vi "GetLeCroy_SaveToFile_25_AVG.vi"(1 "File Array":string[](array[string]), 2 "lines per plane":i32, 5 "Digitizer Settings":T1={"Digitizer delay (us) "=0.0, "rf points per line"=2048, "lines per plane"=128, "Samp Rate (Hz)"=100000000.0, "Additional dig delay (us)"=0.0, "Voltage Scale"=0.4, "Pre-Looks"=0, "Offset delay (us)"=0.0, "bits A/D"=8, "Avg Num"=1, "DigTimeOut"=5.0, "Rel Dig Delay"=0.0, "Dig Ch"=0, "LeCroyCluster"={"LeCroy Channels"=[TRUE, FALSE, FALSE, FALSE], "LC read pt offset"=0.0, "Sweep Avg"=FALSE}, "Main Digitizer"=enum."NI Digitizer", "Dig Config"=enum."Single channel", "Digitizer ID Cluster"={"Acqiris/Alazar/SP ID"=[], "NI Instr Handles"=[], "LeCroy VISA"="", "GaGe Handle"={"Handle"=0, "Sample size"=0, "Resolution"=0, "Offset"=0, "Channels"=0, "Boards"=0}, "ATS Ref"="ATS9350", "Acqiris Address"=["PCI::INSTR0"], "ADQRef"=refnum, "adq_cu_ptr"=refnum}, "Trigger Settings"={"Trig Source"=1, "Trig Coupling"=0, "Trig Slope"=0, "Level (mV)"=1500.0}, "Bulk Acq"=FALSE, "Bulk Start Indexes"=[], "Data Ref RF"=refnum, "NI ID/Channel"=[], "Total Dig CH"=1, "Xtra Ann Trig delay (us)"=10.0, "Fix Z Delay?"=FALSE, "One Way Transmission?"=FALSE, "Data Ref Log"=refnum} {"Trigger Settings"."Trig Slope" items=["Positive", "Negative"]; "Trigger Settings"."Level (mV)" format="%.2f"; "Trigger Settings"."Trig Coupling" items=["DC 1 MOhm", "AC 1 MOhm", "DC 50 Ohm", "AC 50 Ohm"]; "Trigger Settings"."Trig Source" items=["Chan 1", "External"]; "Rel Dig Delay" format="%.2f"; "DigTimeOut" format="%.2f"; "Avg Num" min=1; "Offset delay (us)" format="%.2f"; "Additional dig delay (us)" format="%.2f"; "Digitizer delay (us)" format="%.2f"}, 11 "errorin":errorcluster) -> (3 "Gain Array":T5(array[cluster]), 6 "VGain (dB)":dbl, 8 "data out":i16[][][](array[numeric]), 14 "Raw VGain (scale)":dbl, 15 "error out":errorcluster)   [LabVIEW 2022 SP3]
uses:
  -DigitizerRoutines/DigitizerSettings.ctl
  -DigitizerRoutines/Digitizer.ctl
  -DigitizerRoutines/DigConfig.ctl
  -DigitizerRoutines/DigitizerID.ctl
  C:/Windows/System32/ADQAPI_dotNet_helper.dll
panel:
  out "read time":u32
  out "save time":u32
  out "Numeric":i32
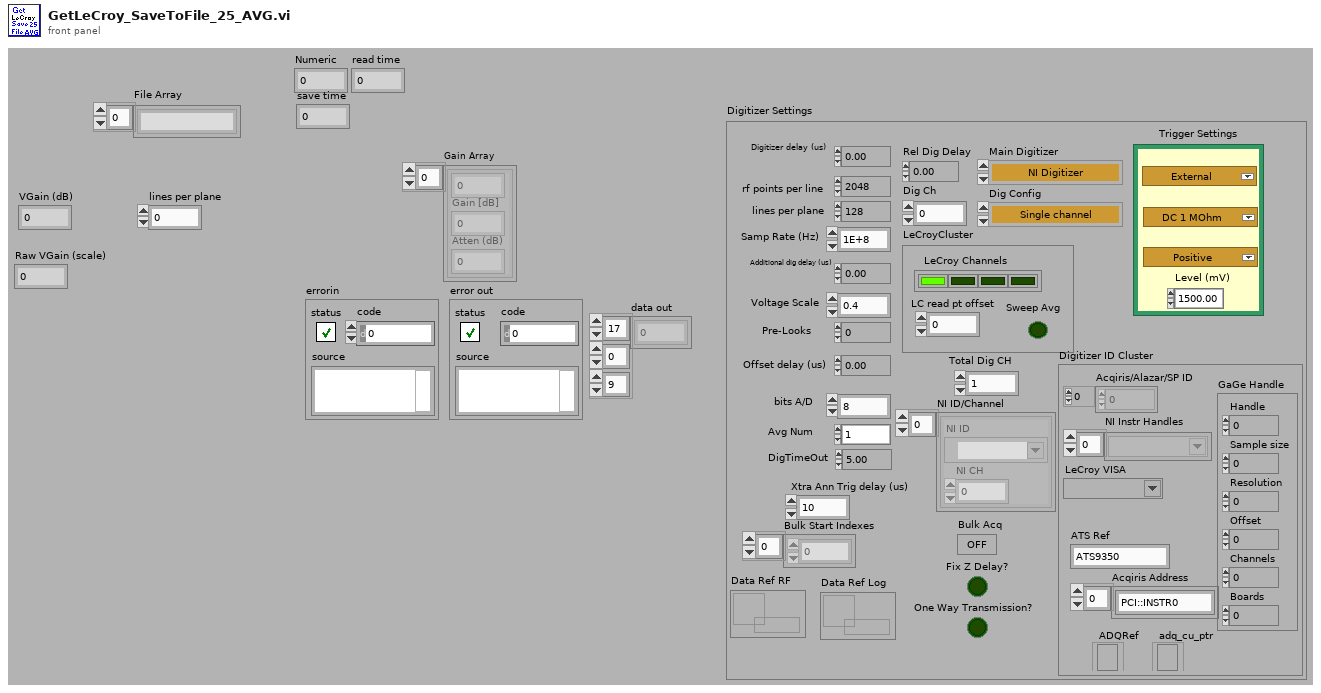
[diagram p1: front panel]
types:
  T1 = typedef "DigitizerSettings.ctl" = cluster{"Digitizer delay (us) ":dbl, "rf points per line":i32, "lines per plane":i32, "Samp Rate (Hz)":dbl, "Additional dig delay (us)":dbl, "Voltage Scale":dbl, "Pre-Looks":i32, "Offset delay (us)":dbl, "bits A/D":i8, "Avg Num":i32, "DigTimeOut":sgl, "Rel Dig Delay":sgl, "Dig Ch":i32, "LeCroyCluster":cluster{"LeCroy Channels":bool[], "LC read pt offset":dbl, "Sweep Avg":bool}, "Main Digitizer":T2, "Dig Config":T3, "Digitizer ID Cluster":T4, "Trigger Settings":cluster{"Trig Source":u16, "Trig Coupling":u16, "Trig Slope":u16, "Level (mV)":dbl}, "Bulk Acq":bool, "Bulk Start Indexes":i32[], "Data Ref RF":refnum<data-value>, "NI ID/Channel":cluster{"NI ID":refnum<k15>, "NI CH":i32}[], "Total Dig CH":i32, "Xtra Ann Trig delay (us)":dbl, "Fix Z Delay?":bool, "One Way Transmission?":bool, "Data Ref Log":refnum<data-value>}
  T2 = typedef "Digitizer.ctl" = enum16{"Acqiris Digitizer", "NI Digitizer", "LeCroy", "GaGe", "AlazarTech", "No Digitizer", "Teledyne"}
  T3 = typedef "DigConfig.ctl" = enum16{"Single channel", "2 Chans w/ 2 Acqiris", "2 Chans w/ 1 Acqiris", "5-CH Pulser New", "5-CH pulser w/ ann array", "5-pass style ann array", "Empty"}
  T4 = typedef "DigitizerID.ctl" = cluster{"Acqiris/Alazar/SP ID":u32[], "NI Instr Handles":refnum<k15>[], "LeCroy VISA":refnum<visa-resource-name>, "GaGe Handle":cluster{"Handle":u32, "Sample size":u32, "Resolution":i32, "Offset":i32, "Channels":u32, "Boards":u32}, "ATS Ref":string, "Acqiris Address":string[], "ADQRef":refnum<k24>, "adq_cu_ptr":refnum<k24>}
  T5 = cluster{sgl, "Gain [dB]  ":sgl, "Atten (dB)":sgl}[]
  T6 = cluster{"wfm":i16[][], "max queue size (-1, unlimited)":i32}
  T7 = cluster{sgl, "Gain [dB]  ":sgl, "Atten (dB)":sgl}
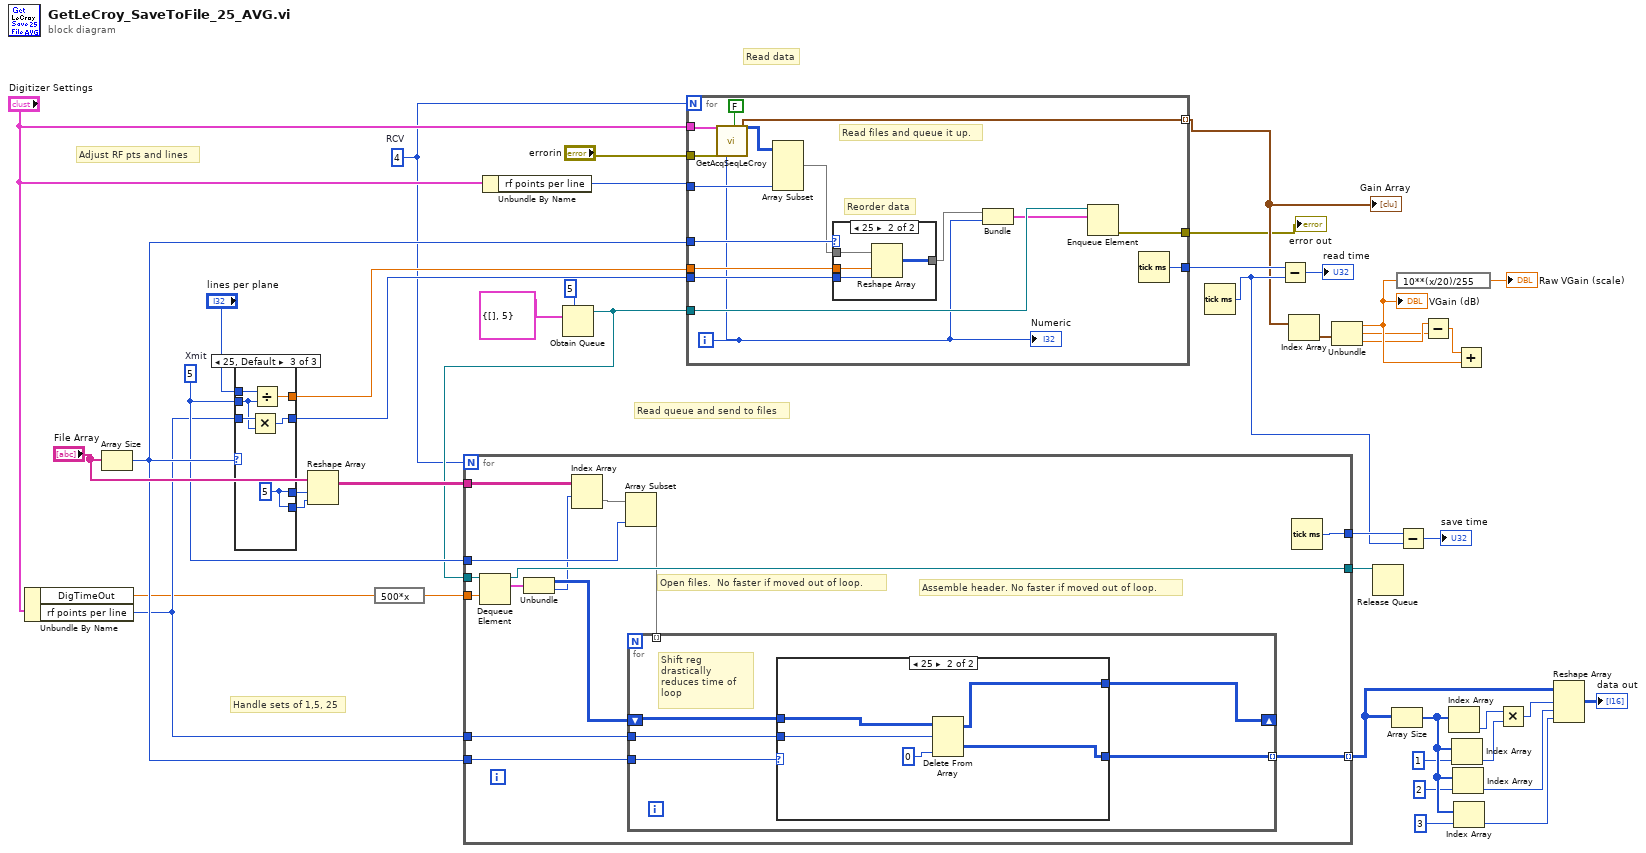
[diagram p0: block diagram]
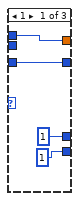
[diagram p3: hidden frame]
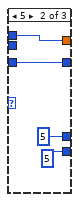
[diagram p4: hidden frame]
diagram:
  w22 = 5  # Xmit
  w3 = 4  # RCV
  # "Read data"
  # "Adjust RF pts and lines"
  # "Handle sets of 1,5, 25"
  # "Read queue and send to files"
  n1 = Unbundle By Name("Digitizer Settings") -> ("DigTimeOut"=w9:sgl, "rf points per line"=w10:i32)
  n2 = Array Size(array="File Array") -> (size(s)=w24:i32)
  n3 = case shown="25, Default" w24 {
    tunnel: [1 5 w58] -> w29
    tunnel: [w47 w51 w54] -> w26
    tunnel: w10 -> [w47 w51 w55]
    tunnel: [w46 w50 w56] -> w27
    tunnel: "lines per plane" -> [w46 w50 w57]
    tunnel: [1 5 w58] -> w28
    tunnel: w22 -> [_ _ w53]
    frame 1 {
    }
    frame 5 {
    }
    frame 25, Default {
      w58 = 5
      n4 = Multiply(x=w55, y=w53) -> (x*y=w54:i32)
      n5 = Divide(x=w57, y=w53) -> (x/y=w56:dbl)
    }
  }
  n6 = Reshape Array("File Array", w29, w28) -> (w23:string[][])
  n7 = expression code="500*x"(w9) -> (w25:sgl)
  n8 = Unbundle By Name("Digitizer Settings") -> ("rf points per line"=w7:i32)
  n9 = Obtain Queue(max queue size (-1, unlimited)=5, element data type=T6 {"wfm"=[], "max queue size (-1, unlimited)"=5}) -> (queue out=w6:refnum<queue>)  [unwired: 3 in, 2 out]
  n10 = for {
    N: w3 -> [_]
    tunnel: w10 -> [w72]
    tunnel: w6 -> [w71]
    tunnel: [w69] -> w31
    tunnel: [w68] -> w35
    tunnel: w24 -> [w67]
    tunnel: w25 -> [w66]
    tunnel: w23 -> [w65]
    tunnel: w22 -> [w63]
    tunnel: [w60] -> w11 mode=indexing
    # "Open files.  No faster if moved out of loop."
    # "Assemble header. No faster if moved out of loop."
    n11 = Dequeue Element(queue=w71, timeout in ms (-1)=w66) -> (queue out=w69:refnum<queue>, element=w70:T6)  [unwired: 1 in, 2 out]
    n12 = Unbundle(w70) -> ("wfm"=w62:i16[][], "max queue size (-1, unlimited)"=w61:i32)
    n13 = Index Array(array=w65, index (row)=w61) -> (element=w64:string[])  [unwired: 1 in]
    n14 = Array Subset(array=w64, length=w63) -> (w59:string[])  [unwired: 1 in]
    n15 = for {
      tunnel: w59 -> [_] mode=indexing
      tunnel: w72 -> [w77]
      tunnel: w67 -> [w75]
      shift-right: [w74] -> _
      shift-left: w62 -> [w76]
      tunnel: [w73] -> w60 mode=indexing
      # "Shift reg drastically reduces time of loop"
      n16 = case shown="25" w75 {
        tunnel: w77 -> [_ w81]
        tunnel: w76 -> [w78 w83]
        tunnel: [w78 w82] -> w74
        tunnel: [w78 w79] -> w73
        frame 5, Default {
        }
        frame 25 {
          n17 = Delete From Array(array=w83, length=w81, index (col)=0 ("index (row)")) -> (deleted portion=w79:i16[][], array with subset deleted=w82:i16[][])  [unwired: 1 in]
        }
      }
    }
    n18 = Tick Count (ms)() -> (millisecond timer value=w68:u32)
  }
  n19 = for {
    N: w3 -> [_]
    tunnel: w6 -> [w99]
    tunnel: [w97] -> w36
    tunnel: [w96] -> w1
    tunnel: w24 -> [w95]
    tunnel: w27 -> [w94]
    tunnel: w26 -> [w93]
    tunnel: w7 -> [w91]
    tunnel: "errorin" -> [w89]
    tunnel: "Digitizer Settings" -> [w87]
    tunnel: [w84] -> w2 mode=indexing
    i -> [w85]
    # "Read files and queue it up."
    # "Reorder data"
    n20 = call "GetAcqSeqLeCroy.vi"("Digitizer Settings"=w87, "errorin"=w89, "Source (0: Channel 1)"=w85, "save?"=FALSE) -> ("Voltage Scale"=w84:T7, "Data Array"=w88:i16[][])  [unwired: 17 in, 5 out]
    n21 = Array Subset(array=w88, length (col)=w91) -> (w90:i16[][])  [unwired: 3 in]
    n22 = case shown="25" w95 {
      tunnel: w93 -> [_ w104]
      tunnel: w90 -> [w100 w103]
      tunnel: [w100 w102] -> w92
      tunnel: w94 -> [_ w101]
      frame 0, Default {
      }
      frame 25 {
        n23 = Reshape Array(w103, w101, w104) -> (w102:i16[][])
      }
    }
    n24 = Bundle(w92, w85) -> (w98:cluster{i16[][], i32})  [unwired: 1 in]
    n25 = Enqueue Element(queue=w99, element=w98) -> (error out=w96:errorcluster)  [unwired: 2 in, 2 out]
    n26 = Tick Count (ms)() -> (millisecond timer value=w97:u32)
    "Numeric" <- w85
  }
  "error out" <- w1
  "Gain Array" <- w2
  n27 = Tick Count (ms)() -> (millisecond timer value=w34:u32)
  n28 = Subtract(x=w36, y=w34) -> (x-y=→"read time":u32)
  n29 = Index Array(array=w2) -> (element=w44:T7)  [unwired: 1 in]
  n30 = Unbundle(w44) -> (w43:sgl, "Gain [dB]"=w41:sgl, "Atten (dB)"=w42:sgl)
  "VGain (dB)" <- w43
  n31 = Release Queue(queue=w31) -> ()  [unwired: 2 in, 3 out]
  n32 = Array Size(array=w11) -> (size(s)=w21:i32[])
  n33 = expression code="10**(x/20)/255"(w43) -> (→"Raw VGain (scale)":sgl)
  n34 = Subtract(x=w35, y=w34) -> (x-y=→"save time":u32)
  n35 = Subtract(x=w42, y=w41) -> (x-y=w40:sgl)
  n36 = Index Array(array=w21) -> (element=w17:i32)  [unwired: 1 in]
  n37 = Index Array(array=w21, index=1) -> (element=w18:i32)
  n38 = Index Array(array=w21, index=2) -> (element=w20:i32)
  n39 = Index Array(array=w21, index=3) -> (element=w19:i32)
  n40 = Add(x=w40, y=w43) -> ()  [unwired: 1 out]
  n41 = Multiply(x=w17, y=w18) -> (x*y=w16:i32)
  n42 = Reshape Array(w11, w16, w20, w19) -> (→"data out":i16[][][])
